vi "roundSD.vi"(1 "digits":dbl=1.0 min=0.0 step=1.0 format="%#_13g", 2 "In":dbl format="%#_13g") -> (0 "Out":dbl format="%#_13g")   [LabVIEW 2015]
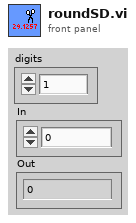
[diagram p1: front panel]
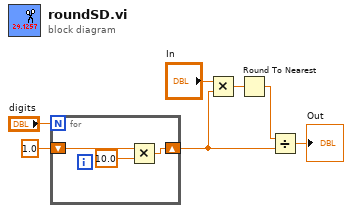
[diagram p0: block diagram]
diagram:
  n1 = for {
    N: "digits" -> [_]
    shift-right: [w9] -> w3
    shift-left: 1.0 -> [w10]
    n2 = Multiply(x=w10, y=10.0) -> (x*y=w9:dbl)
  }
  n3 = Multiply(x="In", y=w3) -> (x*y=w7:dbl)
  n4 = Round To Nearest(number=w7) -> (nearest integer value=w6:dbl)
  n5 = Divide(x=w6, y=w3) -> (x/y=→"Out":dbl)
